vi "Test.vi"() -> ()   [LabVIEW 2015]
panel:
  out "General Settings:Timeout Value":u32
  in  "write buffer":string="*IDN?"
  out "read buffer":string
  out "Interface Information:Interface Type":u16(ring)=1 items=["GPIB"=1, "VXI"=2, "GPIB-VXI"=3, "Serial"=4, "PXI"=5, "TCPIP"=6, "USB"=7, "FireWire"=9]
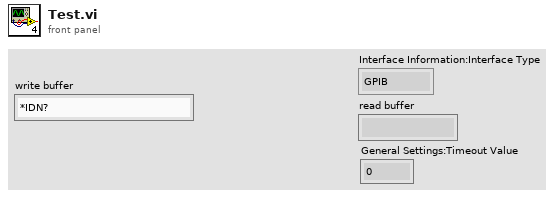
[diagram p1: front panel]
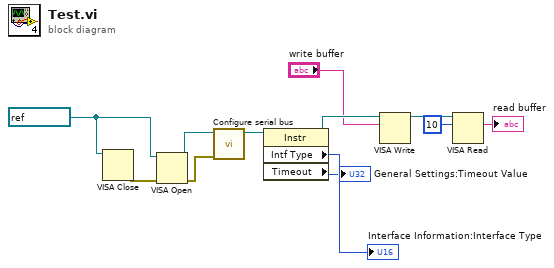
[diagram p0: block diagram]
diagram:
  w2 = refnum<visa-resource-name> "COM4" ("reference")
  n1 = VISA Close(VISA resource name=w2) -> (error out=w5:errorcluster)  [unwired: 1 in]
  n2 = VISA Open(error in (no error)=w5, VISA resource name=w2) -> (VISA resource name=w3:refnum<visa-resource-name>, error out=w4:errorcluster)  [unwired: 3 in]
  n3 = call "Configure serial bus.vi"("Error In"=w4, "VISA resource name"=w3) -> ("VISA resource name 2"=w7:refnum<visa-resource-name>)  [unwired: 7 in, 2 out]
  n4 = property class="Instr"(reference=w7) -> (reference out=w11:refnum<visa-resource-name>, "Intf Type"=→"Interface Information:Interface Type":u16, "Timeout"=→"General Settings:Timeout Value":u32)  [unwired: 1 in, 1 out]
  n5 = VISA Write(VISA resource name=w11, write buffer="write buffer") -> (VISA resource name out=w10:refnum<visa-resource-name>)  [unwired: 1 in, 2 out]
  n6 = VISA Read(VISA resource name=w10, byte count=u32 10) -> (read buffer=→"read buffer":string)  [unwired: 1 in, 3 out]
